vi "Write INI Tokens and VI Tags.vi"(8 "error in (no error)":errorcluster, 11 "Data in":T1={"Class"={"Ants"=refnum, "Layer"=refnum, "Templates"=refnum, "Icon"=refnum, "Glyph"=refnum, "Settings"=refnum, "Tools"=refnum}, "Ref"={"Add Layer"=refnum, "Remove Layer"=refnum, "Line Text"=[], "Body Text Spec"=refnum, "DNL_Font"=refnum, "glyph path str"=refnum, "templates path str"=refnum, "Arrow Up"=refnum, "Arrow Down"=refnum, "IE VI Ref"=refnum, "Glyphs tree"=refnum, "Templates tree"=refnum, "Layer Icon Text"=refnum, "Layer Template"=refnum, "Clipboard"=refnum, "BW icon in"=refnum, "Color icon in"=refnum, "Layer Clust"=refnum, "Body Text"=refnum, "DNL_Framework Templates"=refnum, "Search Templates"=refnum, "TextMarker"=refnum, "Tab Control"=refnum, "Search Glyphs"=refnum, "Line Color"=refnum, "DNL_Glyphs []"=refnum, "Fill Color"=refnum, "Tools"=refnum, "Glyphs tree"=refnum, "Icon"=refnum, "Preview"=refnum, "Ants"=refnum, "Terminals"=refnum, "menu reference"=refnum, "LayerNames"=[], "GlyphLoadAnimation"=refnum, "TemplateLoadAnimation"=refnum, "refreshGlyphs"=refnum, "refreshTemplates"=refnum}, "Support"={"AntsRect"={"left"=0, "top"=0, "right"=0, "bottom"=0}, "Mouse Move Coords"={"Horizontal"=0, "Vertical"=0}, "Mouse Down Coords"={"Horizontal"=0, "Vertical"=0}, "Temp Coord"={"Horizontal"=0, "Vertical"=0}, "Action"=enum."Default", "Edge Color"=4914962, "Fill Color"=16860, "Mouse Down?"=FALSE, "Draft Mode?"=FALSE, "Temp Icon"=bytes[3102], "CTRL Pressed"=FALSE, "Move Selection?"=FALSE, "AntsRect Orig"={"left"=0, "top"=0, "right"=0, "bottom"=0}, "Text"="", "TM Set?"=FALSE, "Mouse inside icon?"=FALSE, "Tool (old value)"=0, "Pencil Move Color"=0, "Swap Colors?"=FALSE, "Shift pressed?"=FALSE}}) -> (0 "error out":errorcluster, 3 "Data out":T1={"Class"={"Ants"=refnum, "Layer"=refnum, "Templates"=refnum, "Icon"=refnum, "Glyph"=refnum, "Settings"=refnum, "Tools"=refnum}, "Ref"={"Add Layer"=refnum, "Remove Layer"=refnum, "Line Text"=[], "Body Text Spec"=refnum, "DNL_Font"=refnum, "glyph path str"=refnum, "templates path str"=refnum, "Arrow Up"=refnum, "Arrow Down"=refnum, "IE VI Ref"=refnum, "Glyphs tree"=refnum, "Templates tree"=refnum, "Layer Icon Text"=refnum, "Layer Template"=refnum, "Clipboard"=refnum, "BW icon in"=refnum, "Color icon in"=refnum, "Layer Clust"=refnum, "Body Text"=refnum, "DNL_Framework Templates"=refnum, "Search Templates"=refnum, "TextMarker"=refnum, "Tab Control"=refnum, "Search Glyphs"=refnum, "Line Color"=refnum, "DNL_Glyphs []"=refnum, "Fill Color"=refnum, "Tools"=refnum, "Glyphs tree"=refnum, "Icon"=refnum, "Preview"=refnum, "Ants"=refnum, "Terminals"=refnum, "menu reference"=refnum, "LayerNames"=[], "GlyphLoadAnimation"=refnum, "TemplateLoadAnimation"=refnum, "refreshGlyphs"=refnum, "refreshTemplates"=refnum}, "Support"={"AntsRect"={"left"=0, "top"=0, "right"=0, "bottom"=0}, "Mouse Move Coords"={"Horizontal"=0, "Vertical"=0}, "Mouse Down Coords"={"Horizontal"=0, "Vertical"=0}, "Temp Coord"={"Horizontal"=0, "Vertical"=0}, "Action"=enum."Default", "Edge Color"=4914962, "Fill Color"=16860, "Mouse Down?"=FALSE, "Draft Mode?"=FALSE, "Temp Icon"=bytes[3102], "CTRL Pressed"=FALSE, "Move Selection?"=FALSE, "AntsRect Orig"={"left"=0, "top"=0, "right"=0, "bottom"=0}, "Text"="", "TM Set?"=FALSE, "Mouse inside icon?"=FALSE, "Tool (old value)"=0, "Pencil Move Color"=0, "Swap Colors?"=FALSE, "Shift pressed?"=FALSE}})   [LabVIEW 2021]
uses:
  <resource>/plugins/NIIconEditor/Controls/INI.ctl
  <vilib>/LabVIEW Icon API/lv_icon/Controls/Font.ctl
  <vilib>/LabVIEW Icon API/lv_icon/Controls/Alignment.ctl
  <resource>/plugins/NIIconEditor/Controls/Font Size.ctl
  <vilib>/LabVIEW Icon API/lv_icon/Controls/BodyText.ctl
  <vilib>/LabVIEW Icon API/lv_icon/Controls/IEColor.ctl
  <resource>/plugins/NIIconEditor/Controls/Tools.ctl
  <resource>/plugins/NIIconEditor/Controls/Pen.ctl
  <resource>/plugins/NIIconEditor/Controls/Line.ctl
  <resource>/plugins/NIIconEditor/Controls/Dropper.ctl
  <resource>/plugins/NIIconEditor/Controls/Fill.ctl
  <resource>/plugins/NIIconEditor/Controls/IERect.ctl
  <resource>/plugins/NIIconEditor/Controls/FRect.ctl
  <resource>/plugins/NIIconEditor/Controls/Circle.ctl
  <resource>/plugins/NIIconEditor/Controls/FCircle.ctl
  <resource>/plugins/NIIconEditor/Controls/Rubber.ctl
  <resource>/plugins/NIIconEditor/Controls/Text.ctl
  <resource>/plugins/NIIconEditor/Controls/Selection.ctl
  <resource>/plugins/NIIconEditor/Controls/Move.ctl
  <resource>/plugins/NIIconEditor/Controls/IE Data.ctl
  <resource>/plugins/NIIconEditor/Class/Ants/Ants.lvclass
  <resource>/plugins/NIIconEditor/Class/FakedArray/FakedArray.lvclass
  <resource>/plugins/NIIconEditor/Class/Icon Library/Glyph.lvclass
  <resource>/plugins/NIIconEditor/Class/Settings/Settings.lvclass
  <resource>/plugins/NIIconEditor/Class/Tools/Tools Paint.lvclass
  <vilib>/LabVIEW Icon API/lv_icon/Classes/Icon/Icon.lvclass
  <resource>/plugins/NIIconEditor/Controls/IE Classes.ctl
  <resource>/plugins/NIIconEditor/Controls/References Cluster.ctl
  <resource>/plugins/NIIconEditor/Controls/SupportClass.ctl
  <vilib>/Utility/miscctls.llb/LVPoint32TypeDef.ctl
  <resource>/plugins/NIIconEditor/Controls/SupportClass_Action.ctl
  <vilib>/LabVIEW Icon API/lv_icon/Classes/Icon Framework/Icon Framework.lvclass
  <vilib>/LabVIEW Icon API/lv_icon/lv_icon.lvlib
  <vilib>/LabVIEW Icon API/lv_icon/Classes/Layer/Layer.lvclass
panel:
  in  "?":T8={"Show Layer Tab?"=FALSE, "Show Terminals?"=FALSE, "Text"={"Font"="", "Alignment"=0, "Size"=0}, "3rd party Templates"={"Store 3rd party Templates?"=FALSE, "Folder Name"=""}, "Merge user layers on commit"=FALSE, "Body Text"={"Line 1 text"="", "Line 2 text"="", "Line 3 text"="", "Line 4 text"="", "Line 1 color"=0, "Line 2 color"=0, "Line 3 color"=0, "Line 4 color"=0, "Body Text Spec"={"Font"="", "Alignment"=0, "Size"=3}, "Center text vertically"=FALSE, "Capitalize Text"=FALSE}, "Fill Color"=0, "Edge Color"=0, "Tab"=0, "Tool"=enum."Ellipse", "Disable Layers?"=FALSE} {"Body Text"."Body Text Spec"."Alignment" items=["left", "center", "right"]; "Text"."Alignment" items=["left", "center", "right"]}
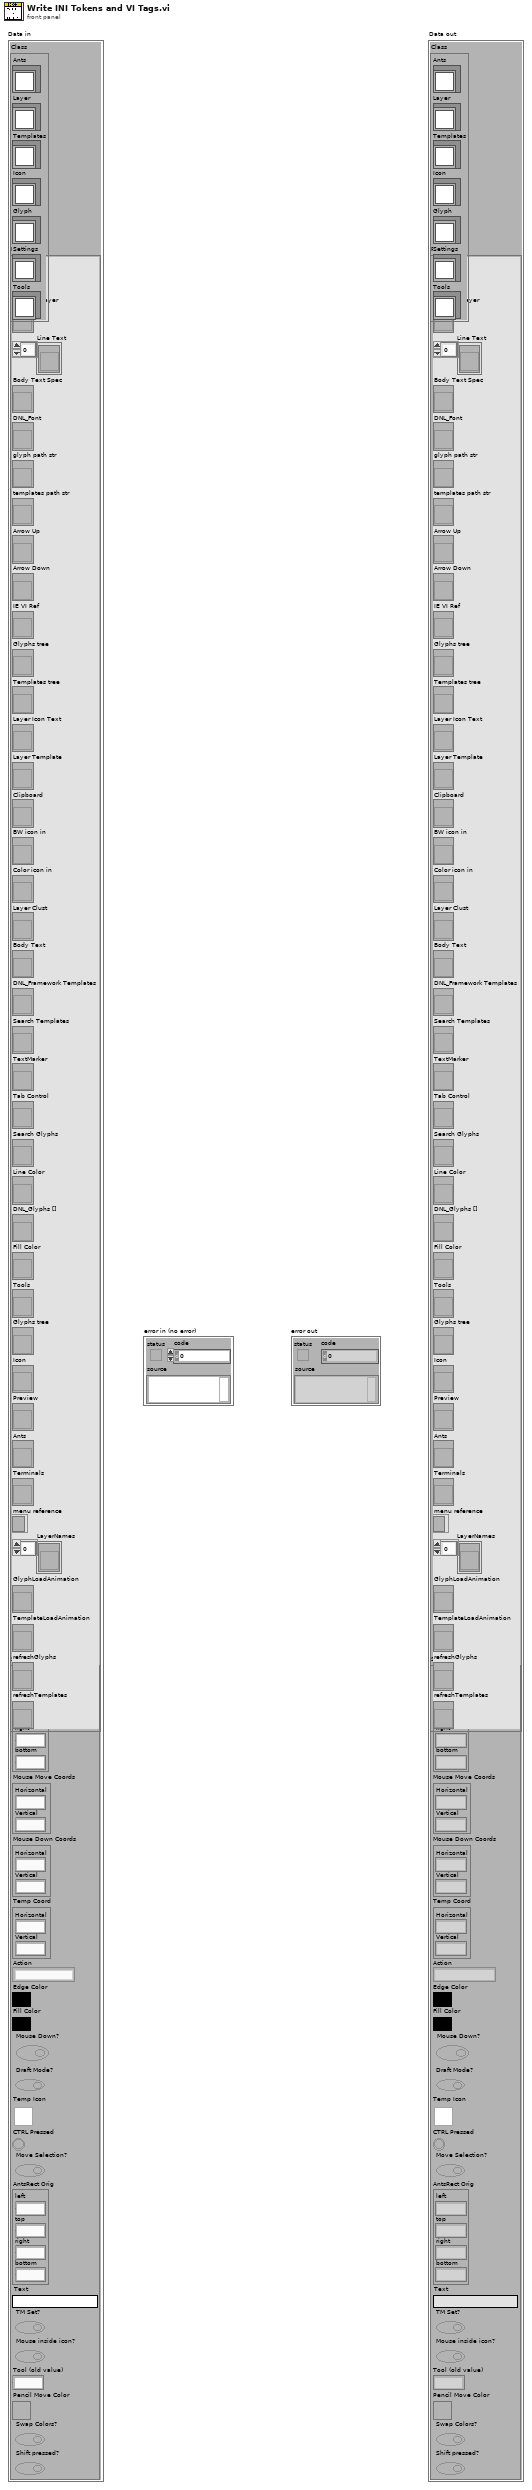
[diagram p1: front panel]
types:
  T1 = typedef "IE Data.ctl" = cluster{"Class":T2, "Ref":T3, "Support":T4}
  T2 = typedef "IE Classes.ctl" = cluster{"Ants":refnum<class "Ants.lvclass">, "Layer":refnum<class "FakedArray.lvclass">, "Templates":refnum<class "FakedArray.lvclass">, "Icon":refnum<class "Icon.lvclass">, "Glyph":refnum<class "Glyph.lvclass">, "Settings":refnum<class "Settings.lvclass">, "Tools":refnum<class "Tools Paint.lvclass">}
  T3 = typedef "References Cluster.ctl" = cluster{"Add Layer":refnum<vi>, "Remove Layer":refnum<vi>, "Line Text":refnum<vi>[], "Body Text Spec":refnum<vi>, "DNL_Font":refnum<vi>, "glyph path str":refnum<vi>, "templates path str":refnum<vi>, "Arrow Up":refnum<vi>, "Arrow Down":refnum<vi>, "IE VI Ref":refnum<vi>, "Glyphs tree":refnum<vi>, "Templates tree":refnum<vi>, "Layer Icon Text":refnum<vi>, "Layer Template":refnum<vi>, "Clipboard":refnum<vi>, "BW icon in":refnum<vi>, "Color icon in":refnum<vi>, "Layer Clust":refnum<vi>, "Body Text":refnum<vi>, "DNL_Framework Templates":refnum<vi>, "Search Templates":refnum<vi>, "TextMarker":refnum<vi>, "Tab Control":refnum<vi>, "Search Glyphs":refnum<vi>, "Line Color":refnum<vi>, "DNL_Glyphs []":refnum<vi>, "Fill Color":refnum<vi>, "Tools":refnum<vi>, "Glyphs tree":refnum<vi>, "Icon":refnum<vi>, "Preview":refnum<vi>, "Ants":refnum<vi>, "Terminals":refnum<vi>, "menu reference":refnum<k9>, "LayerNames":refnum<vi>[], "GlyphLoadAnimation":refnum<vi>, "TemplateLoadAnimation":refnum<vi>, "refreshGlyphs":refnum<vi>, "refreshTemplates":refnum<vi>}
  T4 = typedef "SupportClass.ctl" = cluster{"AntsRect":cluster{"left":i16, "top":i16, "right":i16, "bottom":i16}, "Mouse Move Coords":T5, "Mouse Down Coords":T5, "Temp Coord":T5, "Action":T6, "Edge Color":T7, "Fill Color":T7, "Mouse Down?":bool, "Draft Mode?":bool, "Temp Icon":picture, "CTRL Pressed":bool, "Move Selection?":bool, "AntsRect Orig":cluster{"left":i16, "top":i16, "right":i16, "bottom":i16}, "Text":string, "TM Set?":bool, "Mouse inside icon?":bool, "Tool (old value)":u32, "Pencil Move Color":u32, "Swap Colors?":bool, "Shift pressed?":bool}
  T5 = typedef "LVPoint32TypeDef.ctl" = cluster{"Horizontal":i32, "Vertical":i32}
  T6 = typedef "SupportClass_Action.ctl" = enum16{"Default", "Move Selection", "Glyph Library", "Tool"}
  T7 = typedef "IEColor.ctl" = u32
  T8 = typedef "INI.ctl" = cluster{"Show Layer Tab?":bool, "Show Terminals?":bool, "Text":cluster{"Font":T9, "Alignment":T10, "Size":T11}, "3rd party Templates":cluster{"Store 3rd party Templates?":bool, "Folder Name":string}, "Merge user layers on commit":bool, "Body Text":T12, "Fill Color":T7, "Edge Color":T7, "Tab":u16, "Tool":T13, "Disable Layers?":bool}
  T9 = typedef "Font.ctl" = string
  T10 = typedef "Alignment.ctl" = u16
  T11 = typedef "Font Size.ctl" = u8
  T12 = typedef "BodyText.ctl" = cluster{"Line 1 text":string, "Line 2 text":string, "Line 3 text":string, "Line 4 text":string, "Line 1 color":u32, "Line 2 color":u32, "Line 3 color":u32, "Line 4 color":u32, "Body Text Spec":cluster{"Font":T9, "Alignment":T10, "Size":u8}, "Center text vertically":bool, "Capitalize Text":bool}
  T13 = typedef "Tools.ctl" = enum32{"Pencil", "Line", "Dropper", "Fill", "Rectangle", "Filled Rectangle", "Ellipse", "Filled Ellipse", "Eraser", "Text", "Select", "Move"}
  T14 = cluster{"LayerIcon":picture, "LayerName":string, "Opacity":u8, "Visibility?":bool}
  T15 = enum32{"Pencil", "Line", "Dropper", "Fill", "Rectangle", "Filled Rectangle", "Ellipse", "Filled Ellipse", "Eraser", "Text", "Select", "Move"}
  T16 = typedef "Icon Editor Invoker Type.ctl" = enum32{"Unknown Icon Source", "VI Icon", "Library Icon (any library type)", "Palette icon", "Icon from App Method"}
  T17 = typedef "Pathes.ctl" = enum16{"Root Path", "Icon Templates", "Icon Templates VI", "Icon Templates Lib", "Glyphs"}
  T18 = typedef "Graphic.ctl" = cluster{"Rectangle":cluster{"left":i16, "top":i16, "right":i16, "bottom":i16}, "Path":path, "Image":picture, "Filter":string, "FileName":string}
  T19 = cluster{"Visibility?":bool, "Opacity":u8, "Visibility?":bool, "Opacity":u8, "Relative Path from 1 to 2":path, "Image":picture, "Layers out":refnum<class "Layer.lvclass">[], "Body Text":T12}
  T20 = enum32{"Templates", "Icon Text", "Glyphs", "Layers"}
  T21 = cluster{"Same Folder Structure?":bool, "Folder Name":string}
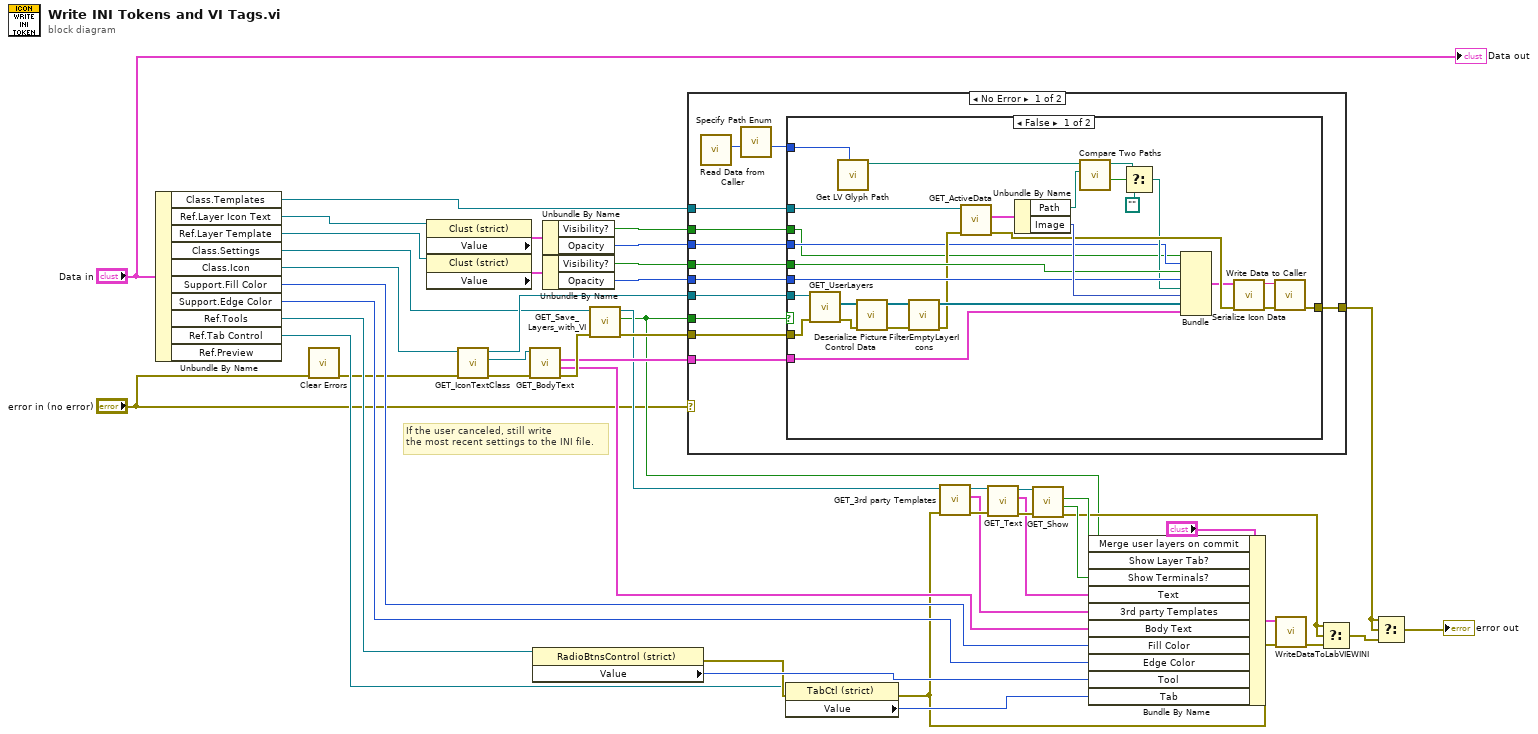
[diagram p0: block diagram]
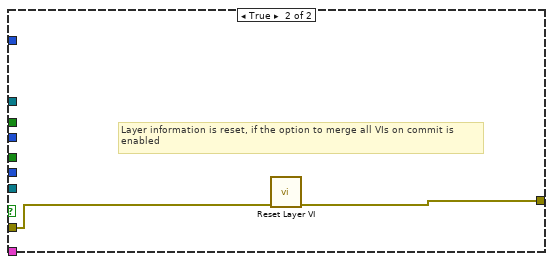
[diagram p2: hidden frame]
diagram:
  # "If the user canceled, still write\nthe most recent settings to the INI file."
  n1 = Unbundle By Name("Data in") -> ("Class.Templates"=w9:refnum<class "FakedArray.lvclass">, "Ref.Layer Icon Text"=w7:refnum<vi>, "Ref.Layer Template"=w15:refnum<vi>, "Class.Settings"=w17:refnum<class "Settings.lvclass">, "Class.Icon"=w16:refnum<class "Icon.lvclass">, "Support.Fill Color"=w14:T7, "Support.Edge Color"=w13:T7, "Ref.Tools"=w12:refnum<vi>, "Ref.Tab Control"=w11:refnum<vi>)  [unwired: 1 out]
  n2 = call <vilib>:"Clear Errors.vi"("error in (no error)"="error in (no error)") -> ("error out"=w2:errorcluster)  [unwired: 5 in, 1 out]
  n3 = property class="Clust (strict)"(reference=w7) -> ("Value"=w8:T14)  [unwired: 1 in, 2 out]
  n4 = property class="Clust (strict)"(reference=w15) -> ("Value"=w21:T14)  [unwired: 1 in, 2 out]
  n5 = call-dynamic "GET_IconTextClass.vi"("error in (no error)"=w2, "Icon.lvclass in"=w16) -> ("error out"=w39:errorcluster, "Icon Framework.lvclass"=w42:refnum<class "Icon Framework.lvclass">, "Icon.lvclass out"=w41:refnum<class "Icon.lvclass">)  [unwired: 7 out]
  n6 = call-dynamic "GET_BodyText.vi"("error in (no error)"=w39, "Icon Framework.lvclass in"=w42) -> ("error out"=w44:errorcluster, "Cleaned Body Text"=w27:T12, "Body Text"=w40:T12)  [unwired: 7 out]
  n7 = property class="RadioBtnsControl (strict)"(reference=w12) -> (error out=w18:errorcluster, "Value"=w28:T15)  [unwired: 1 in, 1 out]
  n8 = Unbundle By Name(w8) -> ("Visibility?"=w5:bool, "Opacity"=w6:u8)
  n9 = Unbundle By Name(w21) -> ("Visibility?"=w19:bool, "Opacity"=w20:u8)
  n10 = call <resource>:"GET_Save_Layers_with_VI.vi"("error in (no error)"=w44, "Settings.lvclass in"=w17) -> ("error out"=w38:errorcluster, "Merge user layers on commit"=w10:bool, "Settings.lvclass out"=w37:refnum<class "Settings.lvclass">)  [unwired: 7 out]
  n11 = case shown="No Error" "error in (no error)" {
    selector: "error in (no error)" -> [_ w89]
    tunnel: [w58 w89] -> w43
    tunnel: w41 -> [w57 _]
    tunnel: w40 -> [w56 _]
    tunnel: w38 -> [w55 _]
    tunnel: w20 -> [w54 _]
    tunnel: w19 -> [w53 _]
    tunnel: w10 -> [w50 _]
    tunnel: w9 -> [w49 _]
    tunnel: w6 -> [w48 _]
    tunnel: w5 -> [w47 _]
    frame No Error {
      n12 = call <resource>:"Read Data from Caller.vi"() -> ("Icon Editor Invoker Type"=w52:T16)  [unwired: 3 in, 8 out]
      n13 = call <resource>:"Specify Path Enum.vi"("Icon Editor Invoker Type"=w52) -> ("Path"=w51:T17)  [unwired: 10 out]
      n14 = case shown="False" w50 {
        tunnel: w57 -> [w85 _]
        tunnel: w55 -> [w79 w88]
        tunnel: w56 -> [w83 _]
        tunnel: [w77 w87] -> w58
        tunnel: w51 -> [w76 _]
        tunnel: w49 -> [w75 _]
        tunnel: w54 -> [w74 _]
        tunnel: w53 -> [w73 _]
        tunnel: w48 -> [w61 _]
        tunnel: w47 -> [w60 _]
        frame False {
          n15 = call-dynamic "GET_UserLayers.vi"("error in (no error)"=w79, "Icon.lvclass in"=w85) -> ("error out"=w70:errorcluster, "All Layers"=w71:refnum<class "Layer.lvclass">[])  [unwired: 8 out]
          n16 = call <vilib>:"Get LV Glyph Path.vi"("Path"=w76) -> ("Requested Path"=w82:path)  [unwired: 2 in, 8 out]
          n17 = call <vilib>:"Deserialize Picture Control Data.vi"("error in (no error)"=w70, "Layers in"=w71) -> ("error out"=w63:errorcluster, "Layers out"=w65:refnum<class "Layer.lvclass">[])  [unwired: 8 out]
          n18 = call <vilib>:"FilterEmptyLayerIcons.vi"("error in (no error)"=w63, "Layers"=w65) -> ("error out"=w62:errorcluster, "Layers out"=w64:refnum<class "Layer.lvclass">[])  [unwired: 8 out]
          n19 = call-dynamic "GET_ActiveData.vi"("error in (no error)"=w62, "FakedArray in"=w75) -> ("error out"=w72:errorcluster, "Path & Icon"=w86:T18)  [unwired: 8 out]
          n20 = Unbundle By Name(w86) -> ("Path"=w81:path, "Image"=w84:picture)
          n21 = call <vilib>:"Compare Two Paths.vi"("Path 2"=w81, "Path 1"=w82) -> ("Path 2 Relative to Path 1?"=w69:bool, "Relative Path from 1 to 2"=w68:path)  [unwired: 1 in, 7 out]
          n22 = Select(t=w68, s=w69, f=path "") -> (s? t:f=w67:path)
          n23 = Bundle("Visibility?"=w60, "Opacity"=w61, "Visibility?"=w73, "Opacity"=w74, "Relative Path from 1 to 2"=w67, "Image"=w84, "Layers out"=w64, "Body Text"=w83) -> (w59:T19)  [unwired: 1 out]
          n24 = call <vilib>:"Serialize Icon Data.vi"("error in"=w72, "Icon data"=w59) -> ("error out"=w78:errorcluster, "data string"=w80:string)  [unwired: 8 out]
          n25 = call <resource>:"Write Data to Caller.vi"("error in (no error)"=w78, "Data"=w80) -> ("error out"=w77:errorcluster)  [unwired: 9 out]
        }
        frame True {
          # "Layer information is reset, if the option to merge all VIs on commit is\nenabled"
          n26 = call <resource>:"Reset Layer VI.vi"("error in (no error)"=w88) -> ("error out"=w87:errorcluster)  [unwired: 10 out]
        }
      }
    }
    frame Error {
    }
  }
  n27 = property class="TabCtl (strict)"(reference=w11, error in=w18) -> (error out=w3:errorcluster, "Value"=w4:T20)  [unwired: 1 out]
  n28 = call-dynamic "GET_3rd party Templates.vi"("error in (no error)"=w3, "Settings.lvclass in"=w37) -> ("error out"=w34:errorcluster, "3rd party Templates"=w26:T21, "Settings.lvclass out"=w36:refnum<class "Settings.lvclass">)  [unwired: 7 out]
  n29 = call-dynamic "GET_Text.vi"("error in (no error)"=w34, "Settings.lvclass in"=w36) -> ("error out"=w33:errorcluster, "Text"=w25:cluster{"Font":T9, "Alignment":T10, "Size":T11}, "Settings.lvclass out"=w35:refnum<class "Settings.lvclass">)  [unwired: 7 out]
  n30 = call-dynamic "GET_Show.vi"("error in (no error)"=w33, "Settings.lvclass in"=w35) -> ("error out"=w22:errorcluster, "Show Terminals?"=w24:bool, "Show LayerTab?"=w23:bool)  [unwired: 7 out]
  n31 = Bundle By Name(cluster="?", "Merge user layers on commit"=w10, "Show Layer Tab?"=w23, "Show Terminals?"=w24, "Text"=w25, "3rd party Templates"=w26, "Body Text"=w27, "Fill Color"=w14, "Edge Color"=w13, "Tool"=w28, "Tab"=w4) -> (w32:T8)
  n32 = call <resource>:"WriteDataToLabVIEWINI.vi"("error in (no error)"=w3, "INI Data"=w32) -> ("error out"=w29:errorcluster)  [unwired: 9 out]
  n33 = Select(t=w22, s=w22, f=w29) -> (s? t:f=w31:errorcluster)
  n34 = Select(t=w43, s=w43, f=w31) -> (s? t:f=→"error out":errorcluster)
  "Data out" <- "Data in"
